vi "Read Intake Current.vi"(8 "Proposed Power":dbl, 10 "CAN Talon SRX Ref":T1={"DeviceStatus"={"status"=FALSE, "code"=0, "source"=""}, "Type"=enum."PWM", "PWM"={"PWM Channel"=enum."PWM 1", "DeadBand"={"Name"="", "maxPositivePwm"=0, "minPositivePwm"=0, "centerPwm"=0, "maxNegativePwm"=0, "minNegativePwm"=0, "angularRange"=0}}, "CAN"={"Device Number"=0, "Control Mode"=enum."Percent VBus", "Semaphore"=refnum, "Max Vout"=12.0, "TalonSRX Control Mode"=enum."Percent VBus"}, "Invert"=FALSE}) -> (1 "Actual Power":dbl, 2 "Reverse Trip?":bool, 3 "Forward Trip?":bool)   [LabVIEW 2015]
uses:
  <vilib>/Rock Robotics/WPI/MotorControl/WPI_MotorControlDeviceRef.ctl
  <vilib>/Rock Robotics/WPI/MotorControl/WPI_MotorControlType.ctl
  <vilib>/Rock Robotics/SystemInterfaces/DIO/FPGA_DIOPWMChannel.ctl
  <vilib>/Rock Robotics/WPI/PWM/WPI_PWMDeadband.ctl
  <vilib>/Rock Robotics/WPI/CAN/Jaguar/SubVIs/WPI_CANJaguar_ControlMode.ctl
  <vilib>/Rock Robotics/WPI/CAN/TalonSRX/WPI_CANTalonSRX_APIControlMode.ctl
  Common Code/Change Detect Boolean.vi
  Common Code/Utilities/TimeManager.vi
  Robot Global Data.vi
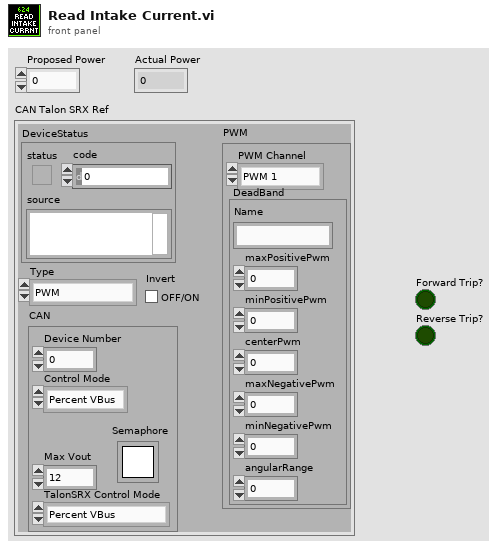
[diagram p1: front panel]
types:
  T1 = typedef "WPI_MotorControlDeviceRef.ctl" = cluster{"DeviceStatus":errorcluster, "Type":T2, "PWM":cluster{"PWM Channel":T3, "DeadBand":T4}, "CAN":cluster{"Device Number":u8, "Control Mode":T5, "Semaphore":T6, "Max Vout":dbl, "TalonSRX Control Mode":T7}, "Invert":bool}
  T2 = typedef "WPI_MotorControlType.ctl" = enum16{"PWM", "CAN", "CANTalonSRX"}
  T3 = typedef "FPGA_DIOPWMChannel.ctl" = enum8{"PWM 0", "PWM 1", "PWM 2", "PWM 3", "PWM 4", "PWM 5", "PWM 6", "PWM 7", "PWM 8", "PWM 9", "PWM MXP 0", "PWM MXP 1", "PWM MXP 2", "PWM MXP 3", "PWM MXP 4", "PWM MXP 5", "PWM MXP 6", "PWM MXP 7", "PWM MXP 8", "PWM MXP 9", "Invalid"}
  T4 = typedef "WPI_PWMDeadband.ctl" = cluster{"Name":string, "maxPositivePwm":i32, "minPositivePwm":i32, "centerPwm":i32, "maxNegativePwm":i32, "minNegativePwm":i32, "angularRange":u16}
  T5 = typedef "WPI_CANJaguar_ControlMode.ctl" = enum8{"Percent VBus", "Current", "Speed", "Position", "Voltage"}
  T6 = typedef "Semaphore RefNum" = refnum<k1>
  T7 = typedef "WPI_CANTalonSRX_APIControlMode.ctl" = enum8{"Percent VBus", "Speed", "Position", "Slave", "Unchanged / Invalid", "Voltage Compensation", "Current", "Motion Profile"}
  T8 = typedef "Dashboard Control Data.ctl" = cluster{"Encoder Control":T9, "Steer PID output":cluster{"output high":dbl, "output low":dbl}, " Steer PID gains":cluster{"proportional gain (Kc)":dbl, "integral time (Ti, min)":dbl, "derivative time (Td, min)":dbl}, "Drivetrain Settings":T10, "Vision Packet":T11, "Info/Command Cluster":T12, "Ball Vision Packet":T13, "Intake Presets":T15, "Intake Encoder Control":T17, "Climb Presets":T18, "Goal Output Range":cluster{"output high":dbl, "output low":dbl}, "Shooter Presets":T19}
  T9 = typedef "Encoder Control.ctl" = cluster{"Right Tick Constant":dbl, "Left Tick Constant":dbl, "Reset?":bool, "Y Dist":cluster{"PID gains":cluster{"proportional gain (Kc)":dbl, "integral time (Ti, min)":dbl, "derivative time (Td, min)":dbl}}, "Y Stop Thresh":dbl, "Y Stop Speed":dbl}
  T10 = typedef "Drivetrain Settings.ctl" = cluster{"Gyro Tolerance":dbl, "Throttle Ramp (ms)":dbl, "Angular rate compensation":bool, "Throttle to Rate Scale":dbl, "Rate compensation gain":dbl, "Kv":dbl, "Ka":dbl, "Feed Forward P":dbl, "Feed Forward D":dbl, "Goal Vision PID gains":cluster{"proportional gain (Kc)":dbl, "integral time (Ti, min)":dbl, "derivative time (Td, min)":dbl}, "Goal Detection Window":dbl}
  T11 = typedef "Goal Vision Packet.ctl" = cluster{"Distance":dbl, "Center X":dbl, "Center Y":dbl, "Found Target?":bool}
  T12 = typedef "Ball Tracking Command Cluster.ctl" = cluster{"Distance to Ball":dbl, "Desired Angle":dbl, "Command":enum16{"Turn to Ball", "Turn to Angle", "Get Distance"}, "Pixels from Center":dbl}
  T13 = typedef "Ball Vision Packet.ctl" = cluster{"Ball Detected?":bool, "Distance to Ball":dbl, "Desired Angle":dbl, "Pixels from Center":dbl, "Tracking mode":T14}
  T14 = typedef "Tracking Mode.ctl" = enum16{"Turn to Ball", "Turn to Angle"}
  T15 = typedef "Intake Presets.ctl" = cluster{"Intake Speed":dbl, "Outake Speed":dbl, "Low Height":dbl, "Half Height":dbl, "Full Height":dbl, "Angle Speed":dbl, "Fast Angle":dbl, "Encoder Scale":dbl, "Load Height":dbl, "Output Range":T16, "Rotation Power Max/Min":dbl, "MaxCurrent":dbl, "Intake Trip Time":dbl, "Idle Height":dbl, "Max Height":dbl, "Reset Encoders?":bool, "PID gains":cluster{"proportional gain (Kc)":dbl, "integral time (Ti, min)":dbl, "derivative time (Td, min)":dbl}}
  T16 = typedef "Drivetrain Output Range.ctl" = cluster{"output high":dbl, "output low":dbl}
  T17 = typedef "IntakeEcoderControl.ctl" = cluster{"Arm Tick Constant":dbl, "Reset?":bool, "Y Dist":cluster{"PID gains":cluster{"proportional gain (Kc)":dbl, "integral time (Ti, min)":dbl, "derivative time (Td, min)":dbl}}, "Y Stop Thresh":dbl, "Y Stop Speed":dbl}
  T18 = typedef "Climb Presets.ctl" = cluster{"Pull Power":dbl, "Unpin Power":dbl, "Time to Hold":dbl}
  T19 = typedef "Shooter Presets.ctl" = cluster{"Batter Shot":T20, "Deep Middle Shot":T20, "Manual Shot":T20, "Left Ticks Per Rotation":dbl, "Right Ticks Per Rotation":dbl, "Low Bar Shot":T20, "Shooter RPM Tolerance":dbl, "IIR Filter Power":dbl, "Trigger Power":dbl, "Fire from Load Delay":i32, "Angle Pot M":dbl, "Angle Pot B":dbl, "Shooter Length":dbl, "String Pot Dist":dbl, "Angle PID gains":cluster{"proportional gain (Kc)":dbl, "integral time (Ti, min)":dbl, "derivative time (Td, min)":dbl}, "Angle Motor Output":cluster{"output high":dbl, "output low":dbl}, "Shooter Angle Tolerance":dbl, "Vision Shoot x^2":dbl, "Vision Shoot x":dbl, "Dist from Axis Cam to Pivot":dbl, "High Goal Center Height":dbl, "Feed Forward Max Accel":dbl, "Feed Forward Kv":dbl, "Backwards Trigger":dbl, "Shot Finish Delay (ms)":dbl, "Angle Max Current":dbl, "Angle Current Trip Time":dbl, "Shooter Intake Angle":dbl, "Vision Shoot c":dbl, "Reset?":bool, "Servo Release Delay":dbl, "Servo Idle Angle":i32, "Servo Hold Angle":i32, "Angle Pot x^2":dbl, "Angle Pot x":dbl, "Angle Pot c":dbl}
  T20 = typedef "Shot Presets.ctl" = cluster{"Left Wheel RPM":dbl, "Right Wheel RPM":dbl, "Angle":dbl}
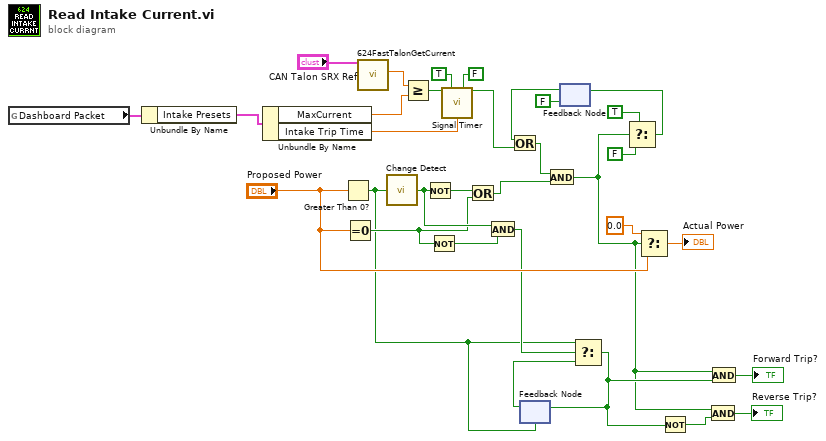
[diagram p0: block diagram]
diagram:
  n1 = global read "Robot Global Data.vi" "Dashboard Packet"() -> (w32:T8)
  n2 = Unbundle By Name(w32) -> ("Intake Presets"=w30:T15)
  n3 = Unbundle By Name(w30) -> ("MaxCurrent"=w29:dbl, "Intake Trip Time"=w27:dbl)
  n4 = Greater Than 0?(x="Proposed Power") -> (x > 0?=w2:bool)
  n5 = Equal To 0?(x="Proposed Power") -> (x = 0?=w4:bool)
  n6 = call "624FastTalonGetCurrent.vi"("CAN Talon SRX Ref"="CAN Talon SRX Ref") -> ("Current"=w31:dbl)  [unwired: 10 in]
  n7 = call-poly "Change Detect.vi"("In"=w2) -> ("Changed?"=w6:bool)
  n8 = Greater Or Equal?(x=w31, y=w29) -> (x >= y?=w28:bool)
  n9 = Not(x=w6) -> (.not. x?=w23:bool)
  n10 = Not(x=w4) -> (.not. x?=w5:bool)
  n11 = call "Signal Timer.vi"("Input"=w28, "Edge"=TRUE, "Interval"=w27, "Pull"=FALSE) -> ("Filtered Output"=w24:bool)  [unwired: 11 in]
  n12 = Or(x=w23, y=w4) -> (x .or. y?=w22:bool)
  n13 = And(x=w6, y=w5) -> (x .and. y?=w3:bool)
  n14 = feedback #1(w2) -> (w12:bool)
  n15 = feedback #2(FALSE) -> (w17:bool)
  n16 = Or(x=w17, y=w24) -> (x .or. y?=w21:bool)
  n17 = And(x=w21, y=w22) -> (x .and. y?=w7:bool)
  n18 = Select(t=w2, s=w3, f=w12) -> (s? t:f=w10:bool)
  n19 = feedback-in #1(w10) -> ()
  n20 = Select(t=TRUE, s=w7, f=FALSE) -> (s? t:f=w18:bool)
  n21 = feedback-in #2(w18) -> ()
  n22 = Select(t=0.0, s=w7, f="Proposed Power") -> (s? t:f=→"Actual Power":dbl)
  n23 = Not(x=w10) -> (.not. x?=w9:bool)
  n24 = And(x=w7, y=w9) -> (x .and. y?=→"Reverse Trip?":bool)
  n25 = And(x=w7, y=w10) -> (x .and. y?=→"Forward Trip?":bool)
